vi "GetRunNumber.vi"(2 "error in (no error)":errorcluster, 3 "Timeout after n trys (default = 100 (10s))":i32=100) -> (0 "error out":errorcluster, 1 "RunNumber":i32)   [LabVIEW 2018]
uses:
  DataPacker/Utilities/PeriodicEnumTypeDef.ctl
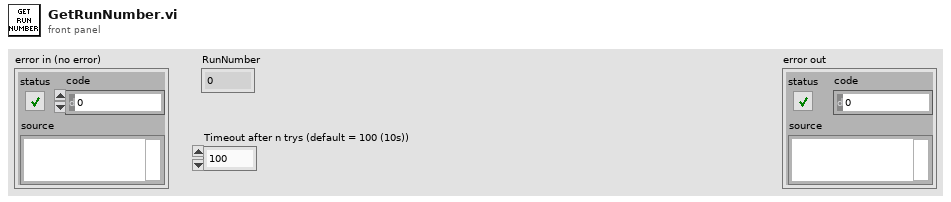
[diagram p1: front panel]
types:
  T1 = typedef "PeriodicEnumTypeDef.ctl" = enum16{"GET_STATUS", "GET_HIST_RATE", "GET_RUNNO", "GET_RUN_START_T", "GET_RUN_STOP_T", "GET_TIME"}
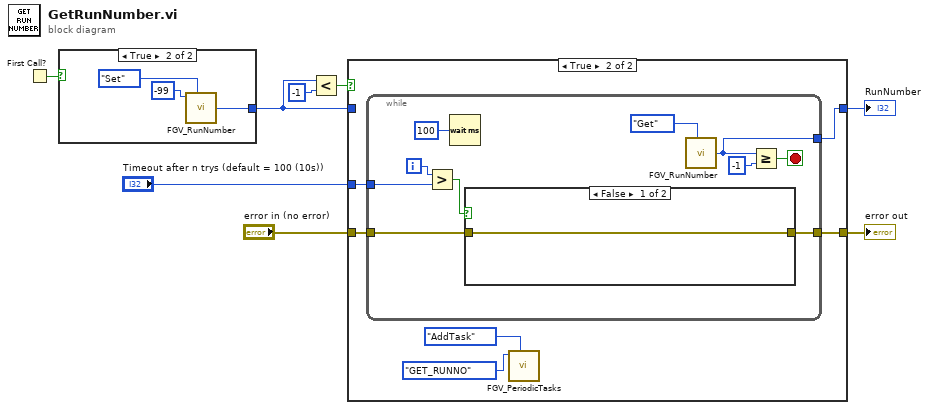
[diagram p0: block diagram]
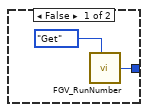
[diagram p2: hidden frame]
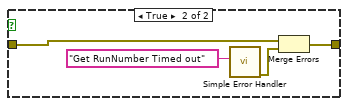
[diagram p4: hidden frame]
diagram:
  n1 = First Call?() -> (First Call?: T/F=w2:bool)
  n2 = case shown="True" w2 {
    tunnel: [w9 w11] -> w1
    frame False {
      n3 = call "FGV_RunNumber.vi"("Enum"=enum16{"Set", "Get"}."Get") -> ("Run Number"=w9:i32)  [unwired: 4 in]
    }
    frame True {
      n4 = call "FGV_RunNumber.vi"("Run Number"=-99, "Enum"=enum16{"Set", "Get"}."Set") -> ("Run Number"=w11:i32)  [unwired: 3 in]
    }
  }
  n5 = Less?(x=w1, y=-1) -> (x < y?=w3:bool)
  n6 = case shown="True" w3 {
    tunnel: [w15 w21] -> w8
    tunnel: w1 -> [w15 _]
    tunnel: "error in (no error)" -> [w14 w20]
    tunnel: [w14 w19] -> w7
    tunnel: "Timeout after n trys (default = 100 (10s))" -> [_ w16]
    frame False {
    }
    frame True {
      n7 = while {
        tunnel: [w24] -> w21
        tunnel: w20 -> [w27]
        tunnel: [w26] -> w19
        tunnel: w16 -> [w25]
        i -> [w29]
        stop <- w22 stop-if-true
        n8 = Greater?(x=w29, y=w25) -> (0:w28:bool)
        n9 = Wait (ms)(milliseconds to wait=u32 100) -> ()  [unwired: 1 out]
        n10 = case shown="False" w28 {
          tunnel: w27 -> [w32 w35]
          tunnel: [w32 w33] -> w26
          frame False {
          }
          frame True {
            n11 = call <vilib>:"Simple Error Handler.vi"("error source (\" \")"="Get RunNumber Timed out" ("error source (\" \")")) -> ("error out"=w34:errorcluster)  [unwired: 4 in, 4 out]
            n12 = Merge Errors(w35, w34) -> (w33:errorcluster)
          }
        }
        n13 = call "FGV_RunNumber.vi"("Enum"=enum16{"Set", "Get"}."Get") -> ("Run Number"=w24:i32)  [unwired: 4 in]
        n14 = Greater Or Equal?(x=w24, y=-1) -> (x >= y?=w22:bool)
      }
      n15 = call "FGV_PeriodicTasks.vi"("MIDAS Commands"=PeriodicEnumTypeDef."GET_RUNNO" ("Enum"), "Task"=enum16{"AddTask", "GetTasks", "ClearTasks"}."AddTask" ("Enum 2")) -> ()  [unwired: 3 in, 1 out]
    }
  }
  "error out" <- w7
  "RunNumber" <- w8
